vi "PID.vi"(8 "Boolean":bool, 11 "Numeric in":dbl) -> (3 "Numeric out":dbl)   [LabVIEW 2018]
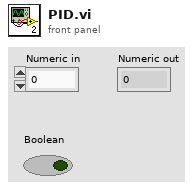
[diagram p1: front panel]
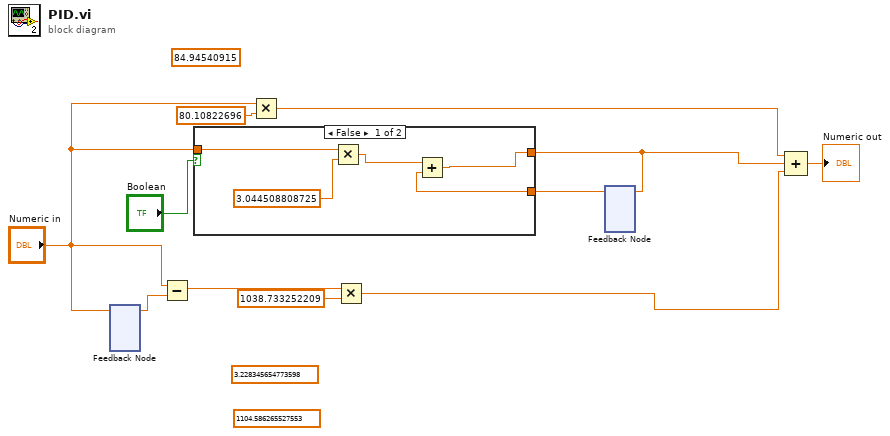
[diagram p0: block diagram]
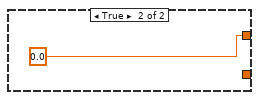
[diagram p2: hidden frame]
diagram:
  (unwired) 1104.586265527553 ("y")
  (unwired) 3.228345654773598 ("x")
  (unwired) 84.94540915 ("y")
  n1 = feedback #1() -> (w11:dbl)  [unwired: 1 in]
  n2 = feedback-in #1("Numeric in") -> ()
  n3 = Subtract(x="Numeric in", y=w11) -> (x-y=w8:dbl)
  n4 = Multiply(x="Numeric in", y=80.10822696) -> (x*y=w3:dbl)
  n5 = Multiply(x=w8, y=1038.733252209) -> (x*y=w1:dbl)
  n6 = feedback #2() -> (w4:dbl)  [unwired: 1 in]
  n7 = case shown="False" "Boolean" {
    tunnel: "Numeric in" -> [w15 _]
    tunnel: [w13 0.0 ("x")] -> w2
    tunnel: w4 -> [w12 _]
    frame False {
      n8 = Multiply(x=w15, y=3.044508808725 ("x")) -> (x*y=w14:dbl)
      n9 = Add(x=w14, y=w12) -> (x+y=w13:dbl)
    }
    frame True {
    }
  }
  n10 = feedback-in #2(w2) -> ()
  n11 = Compound Arithmetic op=ADD(w3, w2, w1) -> (→"Numeric out":dbl)
